vi "Test Express.vi"() -> ()   [LabVIEW 2020]
uses:
  <vilib>/Utility/traverseref.llb/TRef TravTarget.ctl
  SM Template.vit
  FlexBlocks.lvlib
  <vilib>/Utility/traverseref.llb/VI Scripting - Traverse.lvlib
panel:
  out "Array":T1(array[cluster])
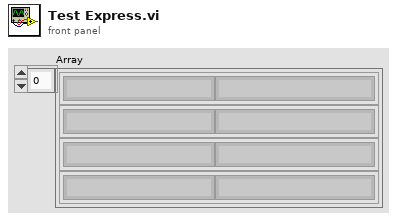
[diagram p1: front panel]
types:
  T1 = cluster{"Label.Text":string, "ClassName":string}[]
  T2 = typedef "TRef TravTarget.ctl" = enum16{"FP", "BD", "Other"}
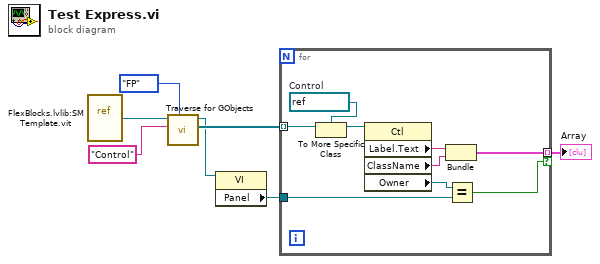
[diagram p0: block diagram]
diagram:
  n1 = vi-ref "FlexBlocks.lvlib:SM Template.vit"() -> (w7:refnum<vi>)
  n2 = call <vilib>:"Traverse for GObjects.vi"("Traverse Target"=TRef_TravTarget."FP", "Class Name"="Control", "VI Refnum"=w7) -> ("References"=w4:refnum<vi>[], "dup VI Refnum"=w2:refnum<vi>)  [unwired: 5 in, 2 out]
  n3 = property class="VI"(reference=w2) -> ("Panel"=w1:refnum<vi>)  [unwired: 1 in, 2 out]
  n4 = for {
    tunnel: w4 -> [w16] mode=indexing
    tunnel: [w11] -> w3 mode=indexing if=w8
    tunnel: w1 -> [w10]
    w15 = refnum<vi> refnum  # Control
    n5 = To More Specific Class(target class=w15, reference=w16) -> (specific class reference=w14:refnum<vi>)  [unwired: 1 in, 1 out]
    n6 = property class="Ctl"(reference=w14) -> ("Label.Text"=w13:string, "ClassName"=w12:string, "Owner"=w9:refnum<vi>)  [unwired: 1 in, 2 out]
    n7 = Bundle("Label.Text"=w13, "ClassName"=w12) -> (w11:cluster{"Label.Text":string, "ClassName":string})  [unwired: 1 in]
    n8 = Equal?(x=w9, y=w10) -> (x = y?=w8:bool)
  }
  "Array" <- w3
